vi "GenClock.vi"() -> ()   [LabVIEW 2013]
uses:
  <vilib>/Utility/error.llb/DialogType.ctl
  <vilib>/DAQmx/write.llb/DAQmx Write (Digital 1D U32 1Chan NSamp).vi
  <vilib>/DAQmx/create/channels.llb/DAQmx Create Channel (CO-Pulse Generation-Frequency).vi
  <vilib>/DAQmx/configure/timing.llb/DAQmx Timing (Implicit).vi
  <vilib>/DAQmx/create/channels.llb/DAQmx Create Channel (DO-Digital Output).vi
  <vilib>/DAQmx/configure/timing.llb/DAQmx Timing (Sample Clock).vi
  <vilib>/DAQmx/miscellaneous.llb/DAQmx Fill In Error Info.vi
  <resource>/objmgr/daqmx.rc
panel:
  in  "Line(s)":tag="Dev1/port0/line0:1"
  in  "Sample Clock Source":tag="PFI0"
  out "Actual Sample Rate":dbl=6000.0 format="%0.2f"
  out "Actual Duty Cycle":dbl=0.5
  out "Actual Frequency":dbl=6000.240009600384
  in  "Duty Cycle":dbl=0.5 format="%.6f"
  in  "Frequency":dbl=6000.0 format="%.6f"
  in  "Output Terminal":tag="/Dev1/PFI12"
  in  "Counter":tag="Dev1/ctr0"
  in  "Stop":bool
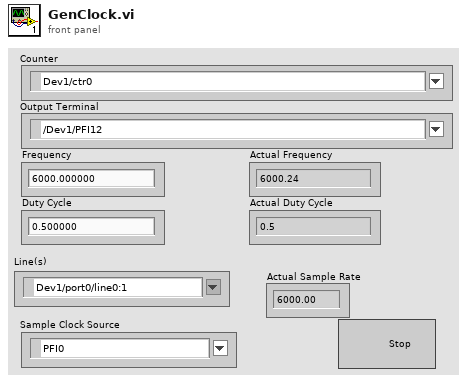
[diagram p1: front panel]
types:
  T1 = typedef "DialogType.ctl" = u16
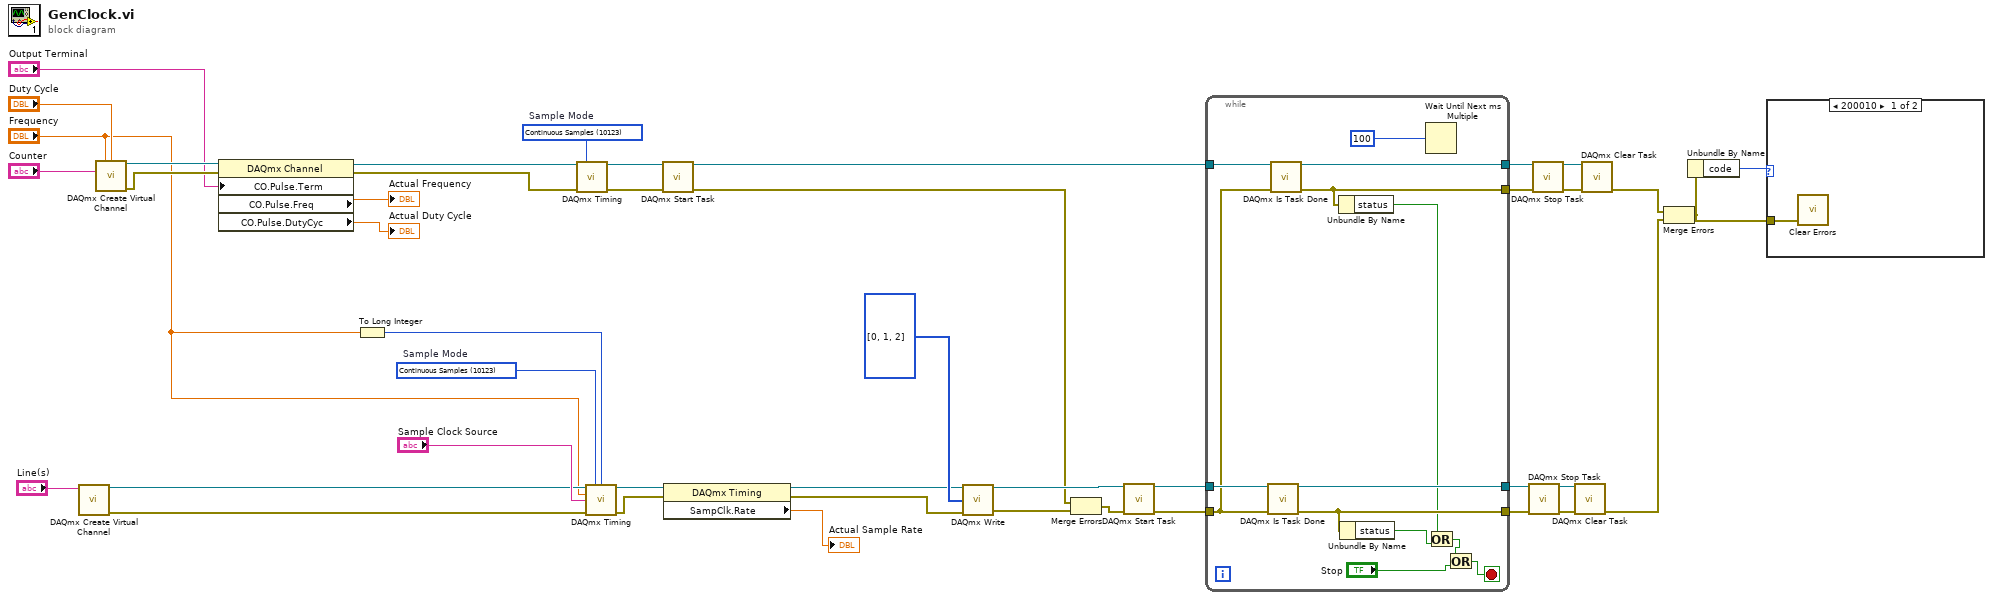
[diagram p0: block diagram]
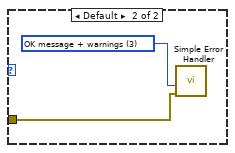
[diagram p2: hidden frame]
diagram:
  w24 = 10123 items=["Finite Samples"=10178, "Continuous Samples"=10123, "Hardware Timed Single Point"=12522]  # Sample Mode
  w44 = 10123 items=["Finite Samples"=10178, "Continuous Samples"=10123, "Hardware Timed Single Point"=12522]  # Sample Mode
  n1 = call-poly <vilib>:"DAQmx Create Virtual Channel.vi"("lines"="Line(s)") -> ("task out"=w26:refnum<k21>, "error out"=w25:errorcluster)  [unwired: 13 in]
  n2 = call-poly <vilib>:"DAQmx Create Virtual Channel.vi"("frequency"="Frequency", "duty cycle"="Duty Cycle", "counter"="Counter") -> ("task out"=w41:refnum<k21>, "error out"=w40:errorcluster)  [unwired: 11 in]
  n3 = property class="DAQmx Channel"(reference=w41, error in=w40, "CO.Pulse.Term"="Output Terminal") -> (reference out=w37:refnum<k21>, error out=w38:errorcluster, "CO.Pulse.Freq"=→"Actual Frequency":dbl, "CO.Pulse.DutyCyc"=→"Actual Duty Cycle":dbl)
  n4 = To Long Integer(number="Frequency") -> (32bit integer=w10:i32)
  n5 = call-poly <vilib>:"DAQmx Timing.vi"("task/channels in"=w37, "sample mode"=w44, "error in"=w38) -> ("task out"=w29:refnum<k21>, "error out"=w28:errorcluster)  [unwired: 11 in]
  n6 = call-poly <vilib>:"DAQmx Timing.vi"("task/channels in"=w26, "sample mode"=w24, "samples per channel"=w10, "rate"="Frequency", "source"="Sample Clock Source", "error in"=w25) -> ("task out"=w23:refnum<k21>, "error out"=w22:errorcluster)  [unwired: 8 in]
  n7 = call <vilib>:"DAQmx Start Task.vi"("task/channels in"=w29, "error in"=w28) -> ("task out"=w43:refnum<k21>, "error out"=w7:errorcluster)  [unwired: 12 in]
  n8 = property class="DAQmx Timing"(reference=w23, error in=w22) -> (reference out=w12:refnum<k21>, error out=w11:errorcluster, "SampClk.Rate"=→"Actual Sample Rate":dbl)
  n9 = call-poly <vilib>:"DAQmx Write.vi"("task/channels in"=w12, "data"=u32[] [0, 1, 2] ("Output Array"), "error in"=w11) -> ("task out"=w19:refnum<k21>, "error out"=w8:errorcluster)  [unwired: 10 in, 1 out]
  n10 = Merge Errors(w7, w8) -> (w6:errorcluster)
  n11 = call <vilib>:"DAQmx Start Task.vi"("task/channels in"=w19, "error in"=w6) -> ("task out"=w18:refnum<k21>, "error out"=w5:errorcluster)  [unwired: 12 in]
  n12 = while {
    tunnel: w43 -> [w57]
    tunnel: [w56] -> w31
    tunnel: [w55] -> w30
    tunnel: w18 -> [w54]
    tunnel: [w53] -> w14
    tunnel: [w52] -> w13
    tunnel: w5 -> [w50]
    stop <- w45 stop-if-true
    n13 = call <vilib>:"DAQmx Is Task Done.vi"("task/channels in"=w54, "error in"=w50) -> ("task out"=w53:refnum<k21>, "error out"=w52:errorcluster)  [unwired: 11 in, 1 out]
    n14 = call <vilib>:"DAQmx Is Task Done.vi"("task/channels in"=w57, "error in"=w50) -> ("task out"=w56:refnum<k21>, "error out"=w55:errorcluster)  [unwired: 11 in, 1 out]
    n15 = Unbundle By Name(w55) -> ("status"=w48:bool)
    n16 = Unbundle By Name(w52) -> ("status"=w49:bool)
    n17 = Wait Until Next ms Multiple(millisecond multiple=u32 100) -> ()  [unwired: 1 out]
    n18 = Or(x=w48, y=w49) -> (x .or. y?=w47:bool)
    n19 = Or(x=w47, y="Stop") -> (x .or. y?=w45:bool)
  }
  n20 = call <vilib>:"DAQmx Stop Task.vi"("task/channels in"=w14, "error in"=w13) -> ("task out"=w16:refnum<k21>, "error out"=w15:errorcluster)  [unwired: 12 in]
  n21 = call <vilib>:"DAQmx Stop Task.vi"("task/channels in"=w31, "error in"=w30) -> ("task out"=w33:refnum<k21>, "error out"=w32:errorcluster)  [unwired: 12 in]
  n22 = call <vilib>:"DAQmx Clear Task.vi"("task in"=w16, "error in"=w15) -> ("error out"=w4:errorcluster)  [unwired: 13 in]
  n23 = call <vilib>:"DAQmx Clear Task.vi"("task in"=w33, "error in"=w32) -> ("error out"=w3:errorcluster)  [unwired: 13 in]
  n24 = Merge Errors(w3, w4) -> (w2:errorcluster)
  n25 = Unbundle By Name(w2) -> ("code"=w1:i32)
  n26 = case shown="200010" w1 {
    tunnel: w2 -> [w58 w59]
    frame 200010 {
      n27 = call <vilib>:"Clear Errors.vi"("error in (no error)"=w58) -> ()  [unwired: 6 in, 1 out]
    }
    frame Default {
      w60 = T1 3 items=["no dialog", "OK message", "continue or stop message", "OK message + warnings", "continue/stop + warnings"] ("type of dialog (OK msg:1)")
      n28 = call <vilib>:"Simple Error Handler.vi"("type of dialog (OK msg:1)"=w60, "error in (no error)"=w59) -> ()  [unwired: 3 in, 5 out]
    }
  }
